vi "img test2.vi"() -> ()   [LabVIEW 2009]
uses:
  <vilib>/vision/NI_Vision_Development_Module.lvlib
panel:
  out "unsigned 8bit integer":u8[][](array[numeric])
  out "Image 3":T1(plugin-control)
  out "Image":T1(plugin-control)
  in  "Range":cluster{"Lower value":sgl, "Upper value":sgl}={"Lower value"=0.0, "Upper value"=100.0} {"Upper value" format="%.2f"; "Lower value" format="%.2f"}
  in  "stop":bool
  in  "Range 2":cluster{"Lower value":sgl, "Upper value":sgl}={"Lower value"=0.0, "Upper value"=100.0} {"Upper value" format="%.2f"; "Lower value" format="%.2f"}
  out "Image 2":T1(plugin-control)
  in  "frame diff":i32
  in  "startign rame":i32
  in  "AVI Path":path=path "C:/Users/Kokum Weeratunga/Desktop/ChongWei vs LinDan (japan open 2010).avi"
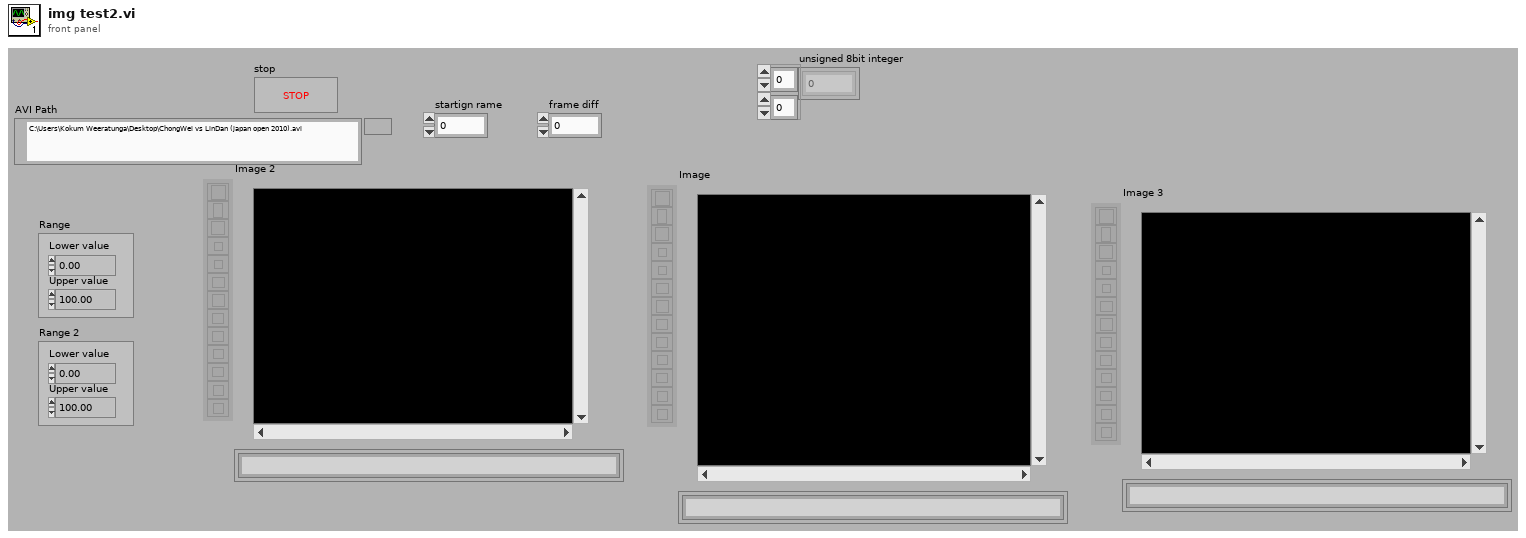
[diagram p1: front panel]
types:
  T1 = typedef "IMAQ Image.ctl" = refnum<image>
  T2 = typedef "Image Type" = u32
  T3 = typedef "AviRefnum.ctl" = refnum<k1>
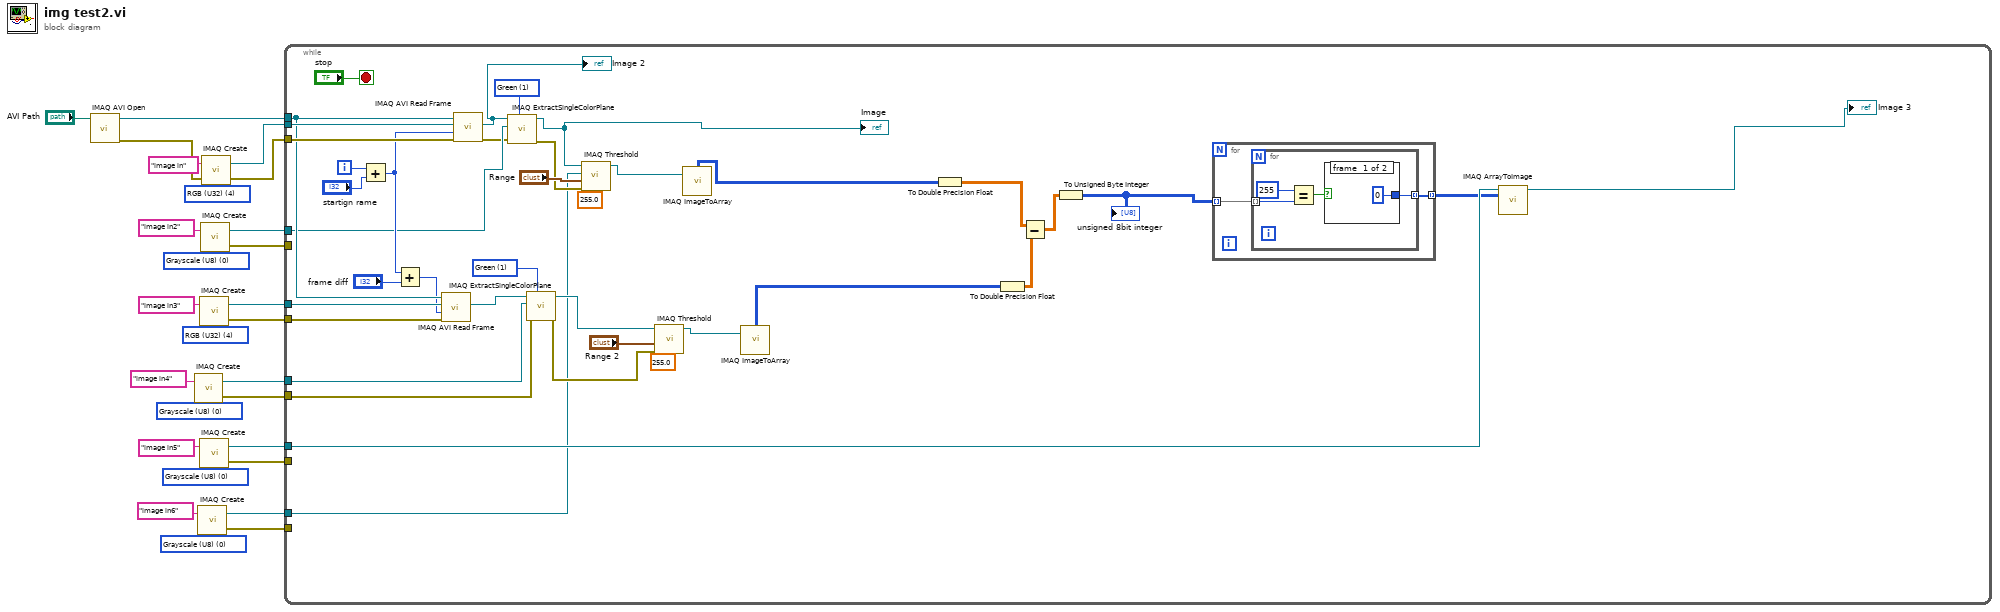
[diagram p0: block diagram]
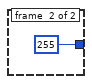
[diagram p2: hidden frame]
diagram:
  w3 = T2 0 items=["Grayscale (U8)", "Grayscale (I16)", "Grayscale (SGL)", "Complex (CSG)", "RGB (U32)", "HSL (U32)", "RGB (U64)", "Grayscale (U16)"] ("Image Type")
  w14 = T2 0 items=["Grayscale (U8)", "Grayscale (I16)", "Grayscale (SGL)", "Complex (CSG)", "RGB (U32)", "HSL (U32)", "RGB (U64)", "Grayscale (U16)"] ("Image Type")
  w12 = T2 4 items=["Grayscale (U8)", "Grayscale (I16)", "Grayscale (SGL)", "Complex (CSG)", "RGB (U32)", "HSL (U32)", "RGB (U64)", "Grayscale (U16)"] ("Image Type")
  w16 = T2 0 items=["Grayscale (U8)", "Grayscale (I16)", "Grayscale (SGL)", "Complex (CSG)", "RGB (U32)", "HSL (U32)", "RGB (U64)", "Grayscale (U16)"] ("Image Type")
  w19 = T2 0 items=["Grayscale (U8)", "Grayscale (I16)", "Grayscale (SGL)", "Complex (CSG)", "RGB (U32)", "HSL (U32)", "RGB (U64)", "Grayscale (U16)"] ("Image Type")
  w22 = T2 4 items=["Grayscale (U8)", "Grayscale (I16)", "Grayscale (SGL)", "Complex (CSG)", "RGB (U32)", "HSL (U32)", "RGB (U64)", "Grayscale (U16)"] ("Image Type")
  n1 = call "IMAQ AVI Open"("AVI Path"="AVI Path") -> ("error out"=w26:errorcluster, "Avi Refnum"=w21:T3)  [unwired: 9 in]
  n2 = call "IMAQ Create"("Image Name"="image in4", "Image Type"=w14) -> ("New Image"=w8:T1, "error out"=w7:errorcluster)  [unwired: 3 in]
  n3 = call "IMAQ Create"("Image Name"="image in6", "Image Type"=w3) -> ("New Image"=w2:T1, "error out"=w1:errorcluster)  [unwired: 3 in]
  n4 = call "IMAQ Create"("Image Name"="image in3", "Image Type"=w12) -> ("New Image"=w10:T1, "error out"=w9:errorcluster)  [unwired: 3 in]
  n5 = call "IMAQ Create"("Image Name"="image in5", "Image Type"=w16) -> ("New Image"=w6:T1, "error out"=w5:errorcluster)  [unwired: 3 in]
  n6 = call "IMAQ Create"("Image Name"="image in2", "Image Type"=w19) -> ("New Image"=w18:T1, "error out"=w17:errorcluster)  [unwired: 3 in]
  n7 = call "IMAQ Create"("Image Name"="image in", "Image Type"=w22, "error in (no error)"=w26) -> ("New Image"=w23:T1, "error out"=w24:errorcluster)  [unwired: 2 in]
  n8 = while {
    tunnel: w24 -> [w66]
    tunnel: w23 -> [w65]
    tunnel: w21 -> [w59]
    tunnel: w18 -> [w49]
    tunnel: w17 -> [_]
    tunnel: w10 -> [w58]
    tunnel: w9 -> [w57]
    tunnel: w8 -> [w45]
    tunnel: w7 -> [w44]
    tunnel: w6 -> [w51]
    tunnel: w5 -> [_]
    tunnel: w2 -> [w31]
    tunnel: w1 -> [_]
    i -> [w55]
    stop <- "stop" stop-if-true
    w32 = 1 items=["Red", "Green", "Blue", "Hue", "Saturation", "Luminance", "Value", "Intensity"] ("Color Plane")
    w46 = 1 items=["Red", "Green", "Blue", "Hue", "Saturation", "Luminance", "Value", "Intensity"] ("Color Plane")
    n9 = Add(x=w55, y="startign rame") -> (x+y=w53:i32)
    n10 = Add(x=w53, y="frame diff") -> (x+y=w56:i32)
    n11 = call "IMAQ AVI Read Frame"("error in (no error)"=w57, "Frame Number"=w56, "Image"=w58, "Avi Refnum"=w59) -> ("Image Out"=w37:T1)  [unwired: 4 in, 3 out]
    n12 = call "IMAQ AVI Read Frame"("error in (no error)"=w66, "Frame Number"=w53, "Image"=w65, "Avi Refnum"=w59) -> ("error out"=w48:errorcluster, "Image Out"=w35:T1)  [unwired: 4 in, 2 out]
    "Image 2" <- w35
    n13 = call "IMAQ ExtractSingleColorPlane"("Color Plane"=w46, "error in (no error)"=w48, "Image Dst"=w49, "Image Src"=w35) -> ("error out"=w47:errorcluster, "Image Dst Out"=w36:T1)  [unwired: 6 in]
    "Image" <- w36
    n14 = call "IMAQ ExtractSingleColorPlane"("Color Plane"=w32, "error in (no error)"=w44, "Image Dst"=w45, "Image Src"=w37) -> ("error out"=w43:errorcluster, "Image Dst Out"=w38:T1)  [unwired: 6 in]
    n15 = call "IMAQ Threshold"("Replace Value"=sgl 255.0, "error in (no error)"=w47, "Range"="Range", "Image Dst"=w31, "Image Src"=w36) -> ("Image Dst Out"=w50:T1)  [unwired: 5 in, 1 out]
    n16 = call "IMAQ Threshold"("Replace Value"=sgl 255.0, "error in (no error)"=w43, "Range"="Range 2", "Image Src"=w38) -> ("Image Dst Out"=w30:T1)  [unwired: 6 in, 1 out]
    n17 = call "IMAQ ImageToArray"("Image"=w50) -> ("Image Pixels (U8)"=w34:u8[][])  [unwired: 3 in, 4 out]
    n18 = call "IMAQ ImageToArray"("Image"=w30) -> ("Image Pixels (U8)"=w29:u8[][])  [unwired: 3 in, 4 out]
    n19 = To Double Precision Float(number=w34) -> (double precision float=w33:dbl[][])
    n20 = To Double Precision Float(number=w29) -> (double precision float=w42:dbl[][])
    n21 = Subtract(x=w33, y=w42) -> (x-y=w41:dbl[][])
    n22 = To Unsigned Byte Integer(number=w41) -> (unsigned 8bit integer=w40:u8[][])
    "unsigned 8bit integer" <- w40
    n23 = for {
      tunnel: w40 -> [w68] mode=indexing
      tunnel: [w67] -> w39 mode=indexing
      n24 = for {
        tunnel: w68 -> [w72] mode=indexing
        tunnel: [w69] -> w67 mode=indexing
        n25 = Equal?(x=u8 255, y=w72) -> (x = y?=w70:bool)
        n26 = case shown="False" w70 {
          tunnel: [u8 0 ("x") u8 255 ("x")] -> w69
          frame #0 {
          }
          frame #1 {
          }
        }
      }
    }
    n27 = call "IMAQ ArrayToImage"("Image Pixels (U8)"=w39, "Image"=w51) -> ("Image Out"=→"Image 3":T1)  [unwired: 8 in, 1 out]
  }
